vi "Temperature Converter.vi"() -> ()   [LabVIEW 2014]
panel:
  out "Converted Temp":dbl
  in  "Temp to Convert":dbl
  in  "Type of Conversion":T1(ring)
  in  "?":bool
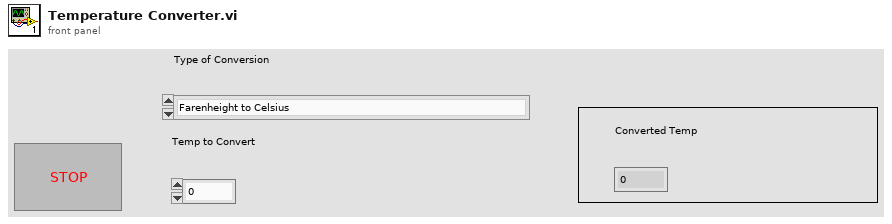
[diagram p1: front panel]
types:
  T1 = enum16{"Farenheight to Celsius", "Celsius to Farenheight", "Celsius to Kelvin", "Farenheight to Kelvin"}
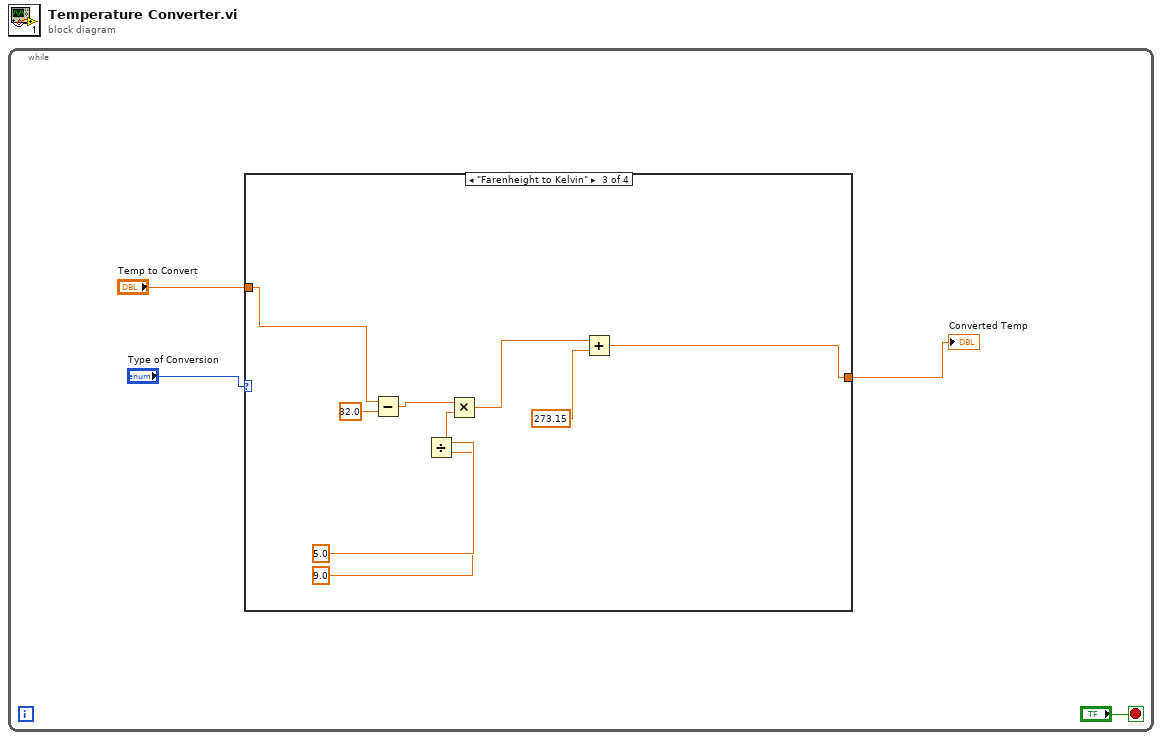
[diagram p0: block diagram]
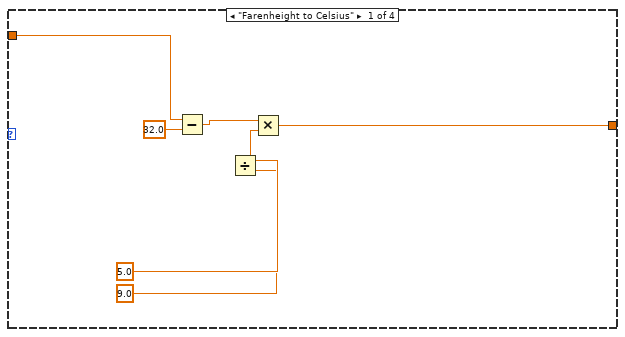
[diagram p2: hidden frame]
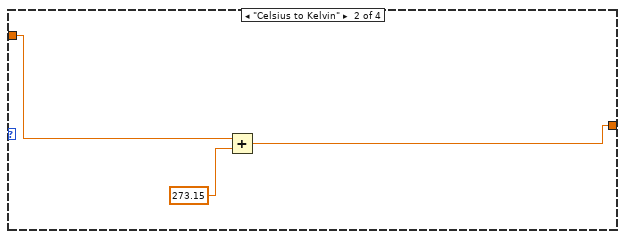
[diagram p3: hidden frame]
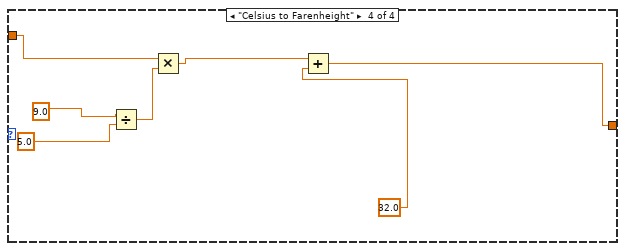
[diagram p4: hidden frame]
diagram:
  n1 = while {
    stop <- "?" stop-if-true
    n2 = case shown="\"Farenheight to Kelvin\"" "Type of Conversion" {
      tunnel: "Temp to Convert" -> [w6 w13 w16 w27]
      tunnel: [w5 w12 w22 w24] -> w1
      frame "Farenheight to Celsius" {
        n3 = Subtract(x=w6, y=32.0) -> (x-y=w8:dbl)
        n4 = Divide(x=5.0 ("x/y"), y=9.0 ("x")) -> (x/y=w7:dbl)
        n5 = Multiply(x=w8, y=w7) -> (x*y=w5:dbl)
      }
      frame "Celsius to Kelvin" {
        n6 = Add(x=w13, y=273.15 ("x+y")) -> (x+y=w12:dbl)
      }
      frame "Farenheight to Kelvin" {
        n7 = Subtract(x=w16, y=32.0) -> (x-y=w18:dbl)
        n8 = Divide(x=5.0 ("x/y"), y=9.0 ("x")) -> (x/y=w17:dbl)
        n9 = Multiply(x=w18, y=w17) -> (x*y=w15:dbl)
        n10 = Add(x=w15, y=273.15) -> (x+y=w22:dbl)
      }
      frame "Celsius to Farenheight" {
        n11 = Divide(x=9.0, y=5.0 ("x/y")) -> (x/y=w28:dbl)
        n12 = Multiply(x=w27, y=w28) -> (x*y=w25:dbl)
        n13 = Add(x=w25, y=32.0) -> (x+y=w24:dbl)
      }
    }
    "Converted Temp" <- w1
  }
